vi "SRQ.vi"(8 "error in (no error)":errorcluster, 9 "SRQ value (0)":i16, 10 "SRQ function (T:set)":bool=TRUE, 11 "VISA resource name":refnum<visa-resource-name>) -> (0 "error out":errorcluster, 1 "display SRQ":i32, 3 "VISA resource name out":refnum<visa-resource-name>)   [LabVIEW 2009, in "Fluke 8840.lvlib"]
doc: "This VI allows the user to enter a new value for the SRQ mask or displays the current value of the SRQ mask. The SRQ mask is an integer value that specifies which conditions will generate a service request."
uses:
  Fluke 8840.lvlib
panel:
  # "set SRQ\ndisplay SRQ"
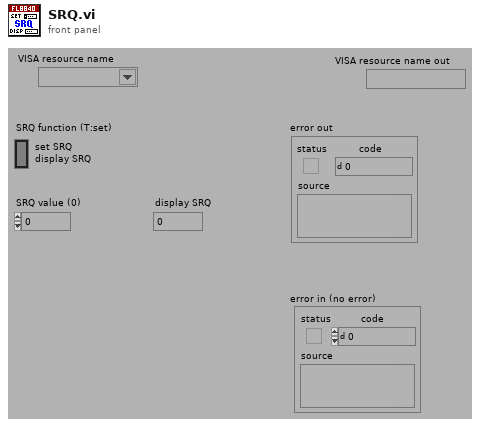
[diagram p1: front panel]
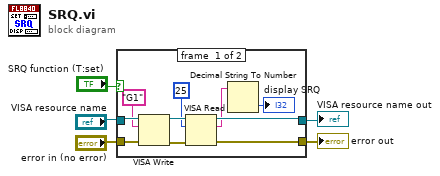
[diagram p0: block diagram]
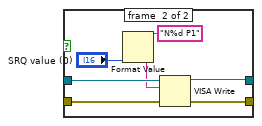
[diagram p2: hidden frame]
diagram:
  n1 = case shown="True" "SRQ function (T:set)" {
    tunnel: "VISA resource name" -> [w15 w22]
    tunnel: "error in (no error)" -> [w14 w21]
    tunnel: [w10 w20] -> w3
    tunnel: [w9 w19] -> w2
    frame #0 {
      n2 = VISA Write(VISA resource name=w15, write buffer="G1", error in (no error)=w14) -> (VISA resource name out=w13:refnum<visa-resource-name>, error out=w12:errorcluster)  [unwired: 1 out]
      n3 = VISA Read(VISA resource name=w13, byte count=u32 25, error in (no error)=w12) -> (VISA resource name out=w10:refnum<visa-resource-name>, read buffer=w7:string, error out=w9:errorcluster)  [unwired: 1 out]
      n4 = Decimal String To Number(string=w7) -> (number=→"display SRQ":i32)  [unwired: 3 out]
    }
    frame #1 {
      n5 = Format Value(format string="N%d P1", value (0)="SRQ value (0)") -> (output string=w16:string)  [unwired: 1 out]
      n6 = VISA Write(VISA resource name=w22, write buffer=w16, error in (no error)=w21) -> (VISA resource name out=w20:refnum<visa-resource-name>, error out=w19:errorcluster)  [unwired: 1 out]
    }
  }
  "error out" <- w2
  "VISA resource name out" <- w3
